vi "Initialize.vi"(7 "Limit Name":string="Setpoint.ch%d.SP", 8 "error in":errorcluster, 9 "Number of Channels":u32=1, 10 "Instance Name":string="PluginName", 11 "Flow Limit in":refnum<class "Flow Limit.lvclass">) -> (0 "error out":errorcluster caption="error in", 3 "Flow Limit out":refnum<class "Flow Limit.lvclass">)   [LabVIEW 2023, in "Flow Limit.lvclass"]
uses:
  Flow Limit.lvclass
  Flow Limit.lvclass/Flow Limit.ctl
  Parents/Limit/Limit.lvclass
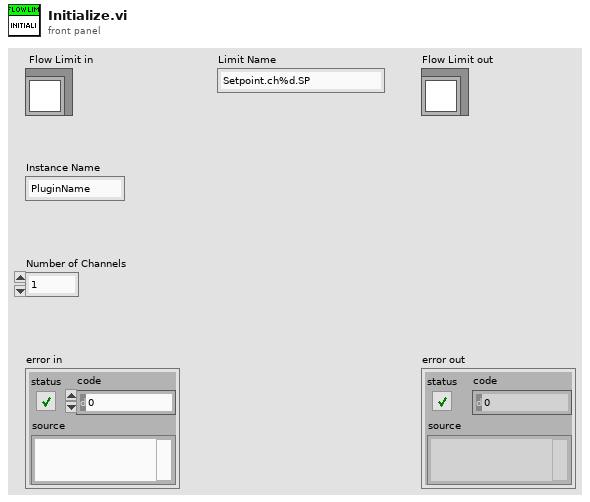
[diagram p1: front panel]
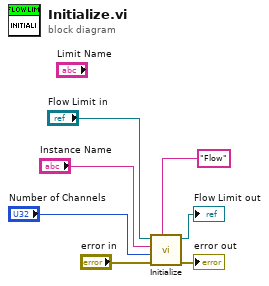
[diagram p0: block diagram]
diagram:
  n1 = call-parent "Initialize.vi"("Limit Name"="Flow", "error in"="error in", "Number of Channels"="Number of Channels", "Instance Name"="Instance Name", "Limit in"="Flow Limit in") -> ("error out"=→"error out":errorcluster, "Limit out"=→"Flow Limit out":refnum<class "Flow Limit.lvclass">)  [unwired: 5 in]
